vi "Agilent SNA Release.vi"(7 "Agilent SNA & SWP":T1, 8 "error in (no error)":errorcluster, 11 "VISA Resource Names":T2) -> (0 "error out":errorcluster {"code" format="%.0x"})   [LabVIEW 2011]
uses:
  TypeDefs/Agilent SNA VISA.ctl
  TypeDefs/Agilent SNA Instrument Info.ctl
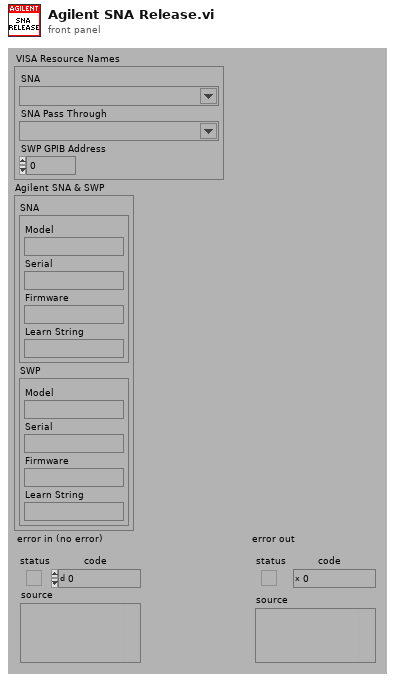
[diagram p1: front panel]
types:
  T1 = typedef "Agilent SNA Instrument Info.ctl" = cluster{"SNA":cluster{"Model":string, "Serial":string, "Firmware":string, "Learn String":string}, "SWP":cluster{"Model":string, "Serial":string, "Firmware":string, "Learn String":string}}
  T2 = typedef "Agilent SNA VISA.ctl" = cluster{"SNA":refnum<visa-resource-name>, "SNA Pass Through":refnum<visa-resource-name>, "SWP GPIB Address":i32}
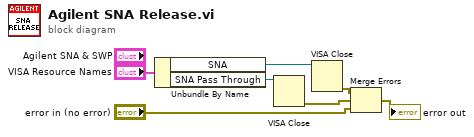
[diagram p0: block diagram]
diagram:
  n1 = Unbundle By Name("VISA Resource Names") -> ("SNA"=w4:refnum<visa-resource-name>, "SNA Pass Through"=w2:refnum<visa-resource-name>)
  n2 = VISA Close(VISA resource name=w2) -> (error out=w1:errorcluster)  [unwired: 1 in]
  n3 = VISA Close(VISA resource name=w4) -> (error out=w7:errorcluster)  [unwired: 1 in]
  n4 = Merge Errors(w7, w1, "error in (no error)") -> (→"error out":errorcluster)
